vi "Laser_COM_old.vi"() -> ()   [LabVIEW 2014]
uses:
  <vilib>/Instr/_visa.llb/Select Event Type.ctl
  <vilib>/Instr/_visa.llb/VISA Configure Serial Port (Instr).vi
panel:
  out "Control ML 2":bool
  out "on/off? 4":bool
  out "f kHz":dbl caption="Темп. модуля" format="%#_g kHz"
  out "7":bool
  out "6":bool
  out "4":bool
  out "5":bool
  out "3":bool
  out "2":bool
  out "1":bool
  out "0":bool
  out "DB25 ML":bool
  out "RS232 ML":bool
  in  "Control ML":bool
  out "on/off? 5":bool
  in  "Laser":bool
  out "Laser EM":bool caption="Излучение включено!"
  out "on/off? 3":bool
  out "on/off? 2":bool
  in  "Send":bool
  in  "write buffer":string caption="Передать команду"
  out "COM_connect":bool
  in  "Connect":bool
  out "SN:":string
  out "ID:":string
  out "Guide  laser":bool
  out "module temp":dbl caption="Темп. модуля" format="%#_g °C"
  in  "Power":dbl(slide) caption="Мощность излучения, %" min=0.0 max=100.0 step=0.5 scale=0.0..100.0 scale format="%#.2g"
  in  "Laser pilot":bool caption="Лазер пилот"
  in  "COM":refnum<visa-resource-name>="COM1" caption="Laser COM-port"
  out "read buffer":string caption="ОТВЕТ:"
  out "error out":errorcluster
  in  "error in (no error)":errorcluster
  # "ID:\n\nSN:"
  # "DB-25"
  # "RS-232"
  # "Блок  управления основным лазером"
  # "Мощьность  излучения, %"
  # "DB-25"
  # "T модуля -"
  # "Пилот Лазер"
  # "Терминал"
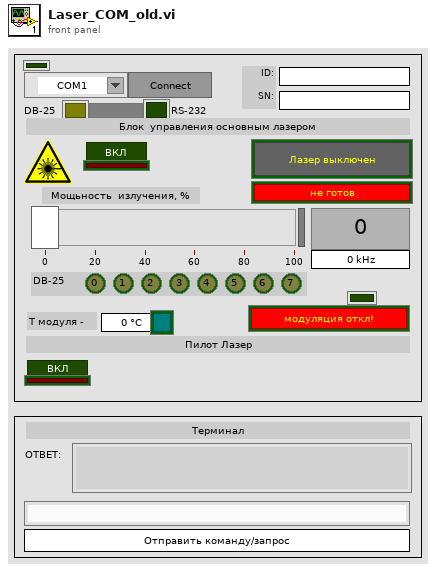
[diagram p1: front panel]
types:
  T1 = typedef "Select Event Type.ctl" = u32
  T2 = cluster{"Control by DB-25":bool, "Control by RS-232":bool, "AuxOFF control by DB-25":bool, "Guide laser control by DB-25":bool, "PRR controlled by Sync line ":bool, "Reserved[1]":bool, "The laser is in Sweep PRR mode":bool, "Modulation control by DB-25":bool, "The laser is in Jump PRR mode":bool, "Reserved[2]":bool, "Bitstream 1 (BS1) mode is active":bool, "Bitstream (BS) mode is active":bool}
  T3 = cluster{"Emergency stop":bool, "External syn frequency on pin 20 is above spec":bool, "External syn frequency on pin 20 is below spec":bool, "Laser ON time (pin 19 HIGH state) is lower spec":bool, "Laser ON time (pin 19 LOW state) is lower spec":bool, "Guide laser":bool, "Reserved [6]":bool, "Reserved [7]":bool, "Laser emission":bool, "Reserved [9]":bool, "Reserved [10]":bool, "Laser emission command was received by RS-232":bool, "Guide laser command was received by RS-232":bool, "24V Main supply voltage is in specified range":bool, "Laser uses 24V housekeeping supply":bool, "Laser uses 5V housekeeping supply":bool, "Manual Prepump is limited by it's max value 10000":bool}
  T4 = cluster{"D0 latched power setting":bool, "D1 latched power setting":bool, "D2 latched power setting":bool, "D3 latched power setting":bool, "D4 latched power setting":bool, "D5 latched power setting":bool, "D6 latched power setting":bool, "D7 latched power setting":bool, "D0 power setting":bool, "D1 power setting":bool, "D2 power setting":bool, "D3 power setting":bool, "D4 power setting":bool, "D5 power setting":bool, "D6 power setting":bool, "D7 power setting":bool, "Latch":bool, "23 AuxOFF Auxiliary Emission OFF":bool, "19 EM Emission Modulation":bool, "22 RG Guide laser control":bool, "20 Sync External Synchronization Input":bool, "18 EE Emission enable":bool, "10 Serial Input":bool, "13 Serial Clock":bool, "16 Laser status":bool, "21 Laser status":bool, "11 Laser status":bool, "12 Serial Output":bool, "24 Serial Enable":bool, "Reserved [29]":bool, "Reserved [30]":bool, "Reserved [31]":bool}
  T5 = cluster{"Module temp is out range":bool, "5V supply voltage is out range":bool, "High rack reflection":bool, "Reserved [1]":bool, "Normal Laser's status":bool, "Laser isn't ready to emmision":bool, "System error":bool, "Reserved [2]":bool}
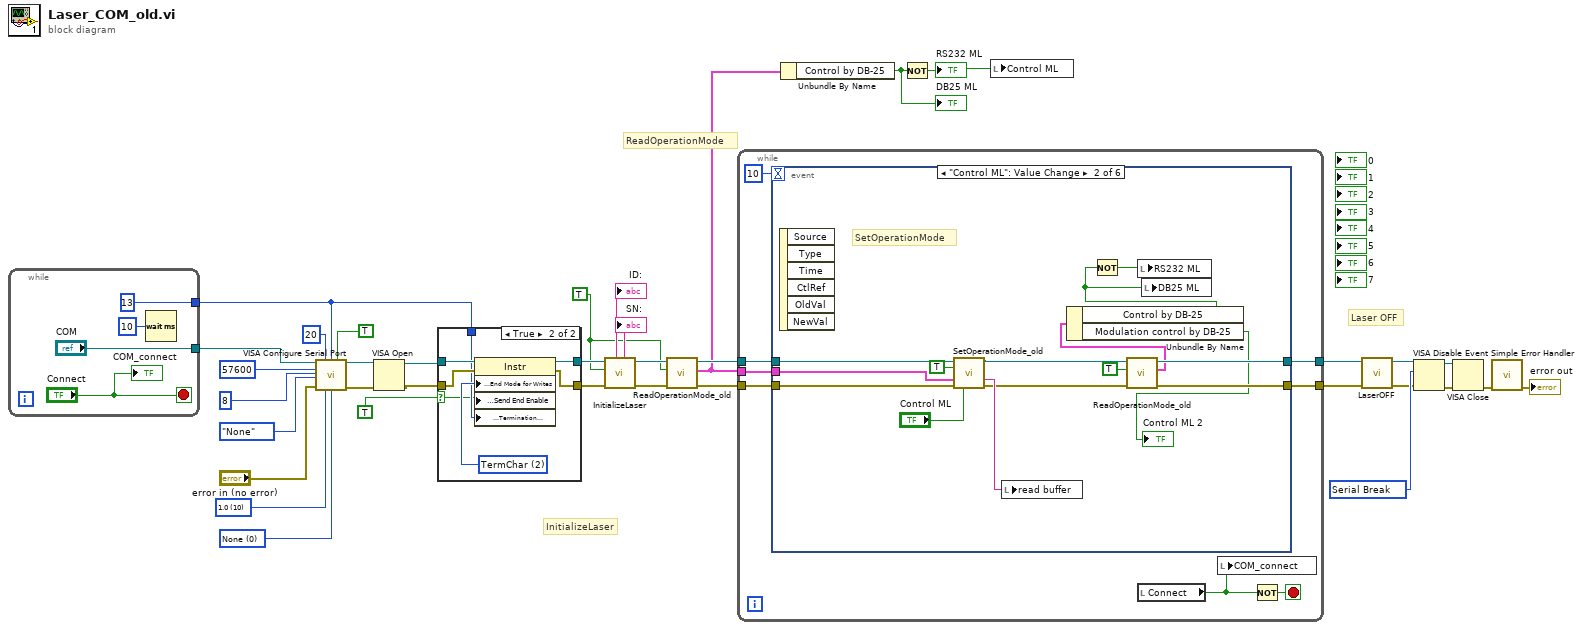
[diagram p0: block diagram]
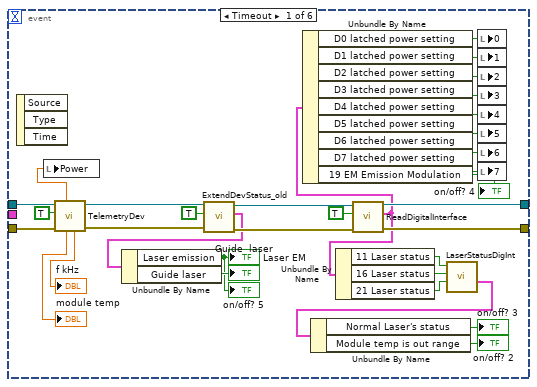
[diagram p2: hidden frame]
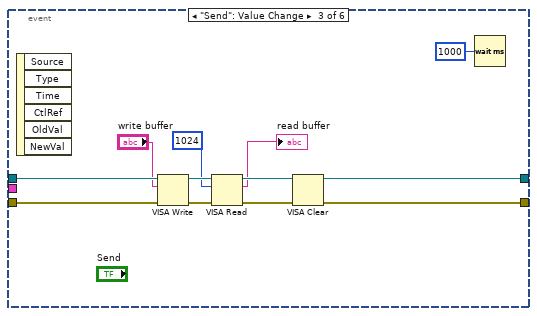
[diagram p3: hidden frame]
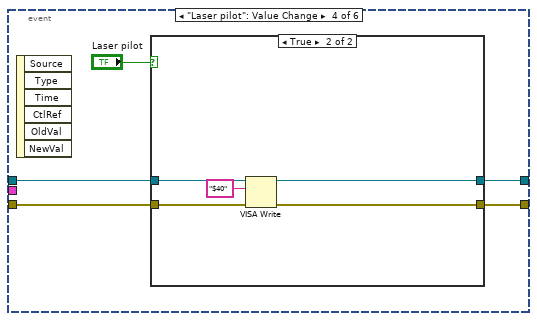
[diagram p4: hidden frame]
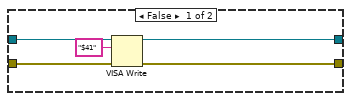
[diagram p5: hidden frame]
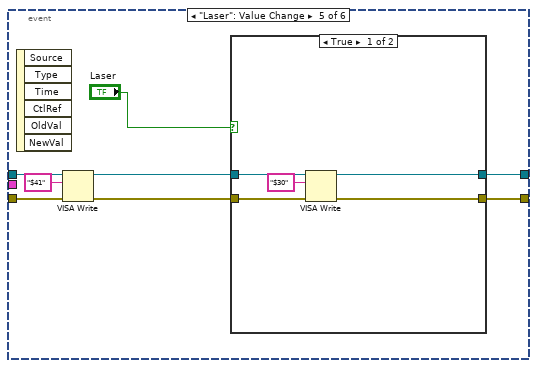
[diagram p6: hidden frame]
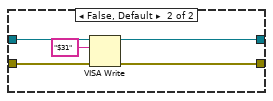
[diagram p7: hidden frame]
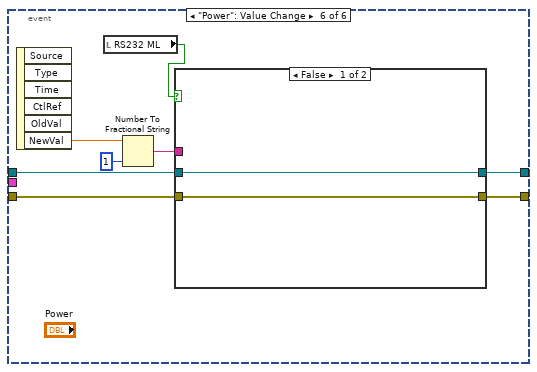
[diagram p8: hidden frame]
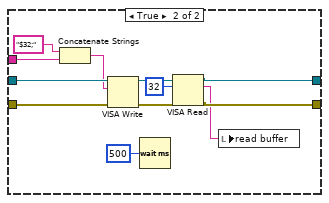
[diagram p9: hidden frame]
diagram:
  w17 = T1 1073684515 items=["Service Request"=1073684491, "Trigger"=3221168138, "Clear"=1073684493, "VXI Signal"=1073684512, "VXI/VME Interrupt"=3221168161, "VXI/VME Sysfail"=1073684509, "VXI/VME Sysreset"=1073684510, "GPIB CIC"=1073684498, "GPIB Talk"=1073684499, "GPIB Listen"=1073684500, "PXI Interrupt"=1073684514, "Serial Break"=1073684515, "Serial TermChar"=1073684516, "Serial CTS"=1073684521, "Serial DSR"=1073684522, "Serial DCD"=1073684524, "Serial RI"=1073684526, "Serial Character"=1073684533, "USB Interrupt"=1073684535, "All Enabled"=1073709055] ("Event Type")
  w22 = u16 0 items=["None", "XON/XOFF", "RTS/CTS", "XON/XOFF & RTS/CTS", "DTR/DSR", "XON/XOFF & DTR/DSR"] ("flow control (0:none)")
  w6 = TRUE
  w29 = u16 10 items=["1.0"=10, "1.5"=15, "2.0"=20] ("stop bits (10: 1 bit)")
  # "Laser OFF"
  # "ReadOperationMode"
  # "InitializeLaser"
  n1 = while {
    tunnel: ["COM"] -> w21
    tunnel: [i16 13 ("term_char")] -> w20
    stop <- "Connect" stop-if-true
    n2 = Wait (ms)(milliseconds to wait=u32 10) -> ()  [unwired: 1 out]
    "COM_connect" <- "Connect"
  }
  n3 = call-poly "VISA Configure Serial Port"("VISA resource name"=w21, "timeout (10sec)"=u32 20, "termination char\n(0xA = '\\n' = LF)"=w20, "Enable Termination\nChar (T)"=TRUE ("Enable Termination\nChar (T)"), "baud rate (9600)"=u32 57600 ("baud rate"), "data bits (8)"=u16 8, "parity (0:none)"=enum16{"None", "Odd", "Even", "Mark", "Space"}."None", "error in (no error)"="error in (no error)", "stop bits (10: 1 bit)"=w29, "flow control (0:none)"=w22) -> ("VISA resource name out"=w32:refnum<visa-resource-name>, "error out"=w31:errorcluster)  [unwired: 4 in]
  n4 = VISA Open(error in (no error)=w31, VISA resource name=w32) -> (VISA resource name=w26:refnum<visa-resource-name>, error out=w27:errorcluster)  [unwired: 3 in]
  n5 = case shown="True" TRUE ("End write with termination character?") {
    selector: TRUE ("End write with termination character?") -> [_ w43]
    tunnel: w26 -> [w41 w49]
    tunnel: w27 -> [w42 w48]
    tunnel: [w41 w47] -> w15
    tunnel: [w42 w46] -> w16
    tunnel: w20 -> [_ w44]
    frame False {
    }
    frame True {
      w45 = u16 2 items=["None", "LastBit", "TermChar", "Break"] ("Serial Settings:Serial End Mode for Writes")
      n6 = property class="Instr"(reference=w49, error in=w48, "Serial Settings:End Mode for Writes"=w45, "Message Based Settings:Send End Enable"=w43, "Message Based Settings:Termination Character"=w44) -> (reference out=w47:refnum<visa-resource-name>, error out=w46:errorcluster)
    }
  }
  n7 = call "InitializeLaser.vi"("error in"=w16, "ON/OFF"=w6, "VISA resource name in"=w15) -> ("error out"=w7:errorcluster, "VISA resource name out"=w8:refnum<visa-resource-name>, "SN:"=→"SN:":string, "Лазер: ID:"=→"ID:":string)  [unwired: 3 in, 2 out]
  n8 = call "ReadOperationMode_old.vi"("error in"=w7, "ON/OFF"=w6, "VISA resource name in"=w8) -> ("error out"=w9:errorcluster, "Operation Mode Status"=w5:T2, "VISA resource name out"=w10:refnum<visa-resource-name>)  [unwired: 5 in, 1 out]
  n9 = while {
    tunnel: w9 -> [w52]
    tunnel: w10 -> [w53]
    tunnel: [w55] -> w12
    tunnel: [w54] -> w11
    tunnel: w5 -> [w51]
    stop <- w57 stop-if-true
    n10 = event shown="[1] \"Control ML\": Value Change" {
      selector: _ -> [_ _ _ _ _ _]
      dyn-events: _ -> [_ _ _ _ _ _]
      timeout: 10 -> [_ _ _ _ _ _]
      tunnel: w53 -> [w89 w105 w117 w122 w139 w158]
      tunnel: w52 -> [w88 w104 w116 w121 w138 w157]
      tunnel: [w82 w94 w111 w120 w137 w154] -> w55
      tunnel: [w81 w95 w110 w119 w136 w153] -> w54
      tunnel: w51 -> [_ w101 _ _ _ _]
      event Timeout {
        n11 = event-data() -> ()  [unwired: 1 in, 3 out]
        n12 = call "TelemetryDev.vi"("error in"=w88, "ON/OFF"=TRUE, "VISA resource name in"=w89) -> ("error out"=w68:errorcluster, "VISA resource name out"=w69:refnum<visa-resource-name>, "Laser PRR, kHz"=→"f kHz":dbl, "module temp"=→"module temp":dbl, "Laser Power,%"=w86:dbl)  [unwired: 4 in]
        n13 = local write "Power"(w86) -> ()
        n14 = call "ExtendDevStatus_old.vi"("error in"=w68, "ON/OFF"=TRUE, "VISA resource name in"=w69) -> ("error out"=w83:errorcluster, "Extend Device Status"=w67:T3, "VISA resource name out"=w84:refnum<visa-resource-name>)  [unwired: 5 in]
        n15 = Unbundle By Name(w67) -> ("Laser emission"=→"Laser EM" →"on/off? 5":bool, "Guide laser"=→"Guide  laser":bool)
        n16 = call "ReadDigitalInterface.vi"("error in"=w83, "ON/OFF"=TRUE, "VISA resource name in"=w84) -> ("error out"=w81:errorcluster, "Extend Device Status"=w63:T4, "VISA resource name out"=w82:refnum<visa-resource-name>)  [unwired: 5 in]
        n17 = Unbundle By Name(w63) -> ("D0 latched power setting"=w70:bool, "D1 latched power setting"=w79:bool, "D2 latched power setting"=w78:bool, "D3 latched power setting"=w77:bool, "D4 latched power setting"=w76:bool, "D5 latched power setting"=w75:bool, "D6 latched power setting"=w74:bool, "D7 latched power setting"=w73:bool, "19 EM Emission Modulation"=→"on/off? 4":bool)
        n18 = Unbundle By Name(w63) -> ("11 Laser status"=w66:bool, "16 Laser status"=w65:bool, "21 Laser status"=w64:bool)
        n19 = call "LaserStatusDigInt.vi"("21"=w64, "16"=w65, "11"=w66) -> ("Laser Status"=w62:T5)  [unwired: 8 in]
        n20 = Unbundle By Name(w62) -> ("Normal Laser's status"=→"on/off? 3":bool, "Module temp is out range"=→"on/off? 2":bool)
        n21 = local write "0"(w70) -> ()
        n22 = local write "1"(w79) -> ()
        n23 = local write "2"(w78) -> ()
        n24 = local write "3"(w77) -> ()
        n25 = local write "4"(w76) -> ()
        n26 = local write "5"(w75) -> ()
        n27 = local write "6"(w74) -> ()
        n28 = local write "7"(w73) -> ()
      }
      event "Control ML": Value Change {
        # "SetOperationMode"
        n29 = event-data() -> ()  [unwired: 1 in, 6 out]
        n30 = call "SetOperationMode_old.vi"("VISA resource name in"=w105, "ON/OFF"=TRUE, "Operation Mode Status"=w101, "error in"=w104, "Laser"="Control ML") -> ("VISA resource name out"=w97:refnum<visa-resource-name>, "Message"=w102:string, "error out"=w96:errorcluster)  [unwired: 8 in]
        n31 = local write "read buffer"(w102) -> ()
        n32 = call "ReadOperationMode_old.vi"("error in"=w96, "ON/OFF"=TRUE, "VISA resource name in"=w97) -> ("error out"=w95:errorcluster, "Operation Mode Status"=w93:T2, "VISA resource name out"=w94:refnum<visa-resource-name>)  [unwired: 5 in, 1 out]
        n33 = Unbundle By Name(w93) -> ("Control by DB-25"=w92:bool, "Modulation control by DB-25"=→"Control ML 2":bool)
        n34 = Not(x=w92) -> (.not. x?=w98:bool)
        n35 = local write "RS232 ML"(w98) -> ()
        n36 = local write "DB25 ML"(w92) -> ()
      }
      event "Send": Value Change {
        n37 = event-data() -> ()  [unwired: 1 in, 6 out]
        n38 = VISA Write(VISA resource name=w117, write buffer="write buffer", error in (no error)=w116) -> (VISA resource name out=w115:refnum<visa-resource-name>, error out=w114:errorcluster)  [unwired: 1 out]
        n39 = VISA Read(VISA resource name=w115, byte count=u32 1024, error in (no error)=w114) -> (VISA resource name out=w113:refnum<visa-resource-name>, read buffer=→"read buffer":string, error out=w112:errorcluster)  [unwired: 1 out]
        n40 = VISA Clear(VISA resource name=w113, error in (no error)=w112) -> (VISA resource name out=w111:refnum<visa-resource-name>, error out=w110:errorcluster)
        n41 = Wait (ms)(milliseconds to wait=u32 1000) -> ()  [unwired: 1 out]
      }
      event "Laser pilot": Value Change {
        n42 = event-data() -> ()  [unwired: 1 in, 6 out]
        n43 = case shown="True" "Laser pilot" {
          tunnel: w122 -> [w127 w132]
          tunnel: w121 -> [w126 w131]
          tunnel: [w124 w129] -> w120
          tunnel: [w123 w128] -> w119
          frame False {
            n44 = VISA Write(VISA resource name=w127, write buffer="$41", error in (no error)=w126) -> (VISA resource name out=w124:refnum<visa-resource-name>, error out=w123:errorcluster)  [unwired: 1 out]
          }
          frame True {
            n45 = VISA Write(VISA resource name=w132, write buffer="$40", error in (no error)=w131) -> (VISA resource name out=w129:refnum<visa-resource-name>, error out=w128:errorcluster)  [unwired: 1 out]
          }
        }
      }
      event "Laser": Value Change {
        n46 = event-data() -> ()  [unwired: 1 in, 6 out]
        n47 = VISA Write(VISA resource name=w139, write buffer="$41", error in (no error)=w138) -> (VISA resource name out=w135:refnum<visa-resource-name>, error out=w134:errorcluster)  [unwired: 1 out]
        n48 = case shown="True" "Laser" {
          tunnel: w135 -> [w144 w149]
          tunnel: w134 -> [w143 w148]
          tunnel: [w142 w147] -> w137
          tunnel: [w141 w146] -> w136
          frame True {
            n49 = VISA Write(VISA resource name=w144, write buffer="$30", error in (no error)=w143) -> (VISA resource name out=w142:refnum<visa-resource-name>, error out=w141:errorcluster)  [unwired: 1 out]
          }
          frame False, Default {
            n50 = VISA Write(VISA resource name=w149, write buffer="$31", error in (no error)=w148) -> (VISA resource name out=w147:refnum<visa-resource-name>, error out=w146:errorcluster)  [unwired: 1 out]
          }
        }
      }
      event "Power": Value Change {
        n51 = event-data() -> ("NewVal"=w152:dbl)  [unwired: 1 in, 5 out]
        n52 = local read "RS232 ML"() -> (w151:bool)
        n53 = Number To Fractional String(number=w152, precision (6)=i16 1) -> (F-format string=w156:string)  [unwired: 2 in]
        n54 = case shown="False" w151 {
          tunnel: w158 -> [w160 w172]
          tunnel: w157 -> [w159 w171]
          tunnel: w156 -> [_ w168]
          tunnel: [w160 w165] -> w154
          tunnel: [w159 w164] -> w153
          frame False {
          }
          frame True {
            n55 = Concatenate Strings("$32;" ("write buffer"), w168) -> (w169:string)
            n56 = VISA Write(VISA resource name=w172, write buffer=w169, error in (no error)=w171) -> (VISA resource name out=w167:refnum<visa-resource-name>, error out=w166:errorcluster)  [unwired: 1 out]
            n57 = Wait (ms)(milliseconds to wait=u32 500) -> ()  [unwired: 1 out]
            n58 = VISA Read(VISA resource name=w167, byte count=u32 32, error in (no error)=w166) -> (VISA resource name out=w165:refnum<visa-resource-name>, read buffer=w163:string, error out=w164:errorcluster)  [unwired: 1 out]
            n59 = local write "read buffer"(w163) -> ()
          }
        }
      }
    }
    n60 = local read "Connect"() -> (w56:bool)
    n61 = local write "COM_connect"(w56) -> ()
    n62 = Not(x=w56) -> (.not. x?=w57:bool)
  }
  n63 = Unbundle By Name(w5) -> ("Control by DB-25"=w1:bool)
  "DB25 ML" <- w1
  n64 = Not(x=w1) -> (.not. x?=w2:bool)
  "RS232 ML" <- w2
  n65 = local write "Control ML"(w2) -> ()
  n66 = call "LaserOFF.vi"("error in"=w11, "VISA resource name in"=w12) -> ("error out"=w3:errorcluster, "VISA resource name out"=w4:refnum<visa-resource-name>)  [unwired: 8 in]
  n67 = VISA Disable Event(8:w3, 10:w17, 11:w4) -> (0:w18:errorcluster, 3:w19:refnum<visa-resource-name>)  [unwired: 1 out]
  n68 = VISA Close(VISA resource name=w19, error in (no error)=w18) -> (error out=w23:errorcluster)
  n69 = call <vilib>:"Simple Error Handler.vi"("error in (no error)"=w23) -> ("error out"=→"error out":errorcluster)  [unwired: 4 in, 4 out]
